vi "Create Adapter.vi"(8 "error in (no error)":errorcluster caption="错误输入（无错误）", 11 "OleDBClass 输入":refnum<class "OleDBClass.lvclass"> caption="DNL_LabVIEW Object in") -> (0 "error out":errorcluster caption="错误输出", 3 "OleDBClass 输出":refnum<class "OleDBClass.lvclass"> caption="DNL_LabVIEW Object out")   [LabVIEW 2012, in "OleDBClass.lvclass"]
uses:
  OleDBClass.lvclass
  OleDBClass.lvclass/OleDBClass.ctl
  System.Data
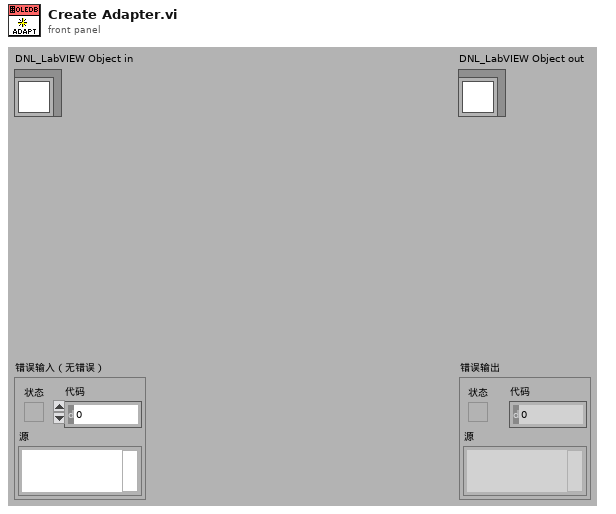
[diagram p1: front panel]
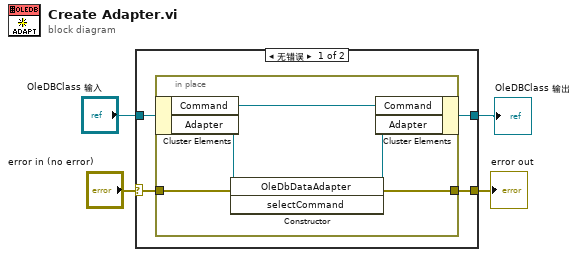
[diagram p0: block diagram]
diagram:
  n1 = case shown="无错误" "error in (no error)" {
    selector: "error in (no error)" -> [w7 w14]
    tunnel: [w5 w14] -> w3
    tunnel: "OleDBClass 输入" -> [w8 w13]
    tunnel: [w6 w13] -> w2
    frame No Error {
      n2 = in-place {
        in-place-border: w7 -> [w10]
        in-place-border: [w9] -> w5
        n3 = in-place-cluster #1(w8) -> ("Command"=w11:refnum<k24>)  [unwired: 1 out]
        n4 = constructor class="OleDbDataAdapter"(error in=w10, "selectCommand"=w11) -> (reference out=w12:refnum<k24>, error out=w9:errorcluster)  [unwired: 2 in, 2 out]
        n5 = in-place-cluster #1("Command"=w11, "Adapter"=w12) -> (w6:refnum<class "OleDBClass.lvclass">)
      }
    }
    frame Error {
    }
  }
  "error out" <- w3
  "OleDBClass 输出" <- w2
